vi "Generate Event.vi"(4 "Error In":errorcluster, 5 "Response Notifier":string, 6 "Data Buffer Depth":i32, 7 "Plugin Name":string) -> (0 "Error Out":errorcluster)   [LabVIEW 2015, in "Set Data Buffer Depth.lvlib"]
uses:
  Set Data Buffer Depth.lvlib
  _typedefs/Event Data.ctl
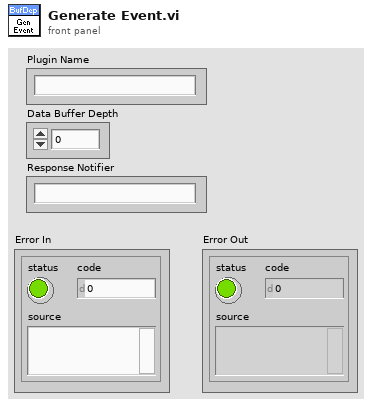
[diagram p1: front panel]
types:
  T1 = typedef "Set Data Buffer Depth.lvlib/Event Data.ctl" = cluster{"Plugin Name":string, "Data Buffer Depth":i32, "Response Notifier":string}
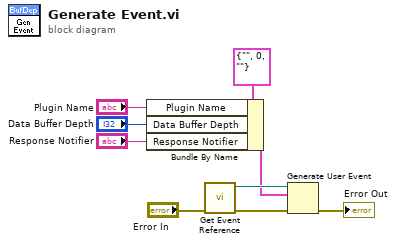
[diagram p0: block diagram]
diagram:
  n1 = Bundle By Name(cluster=T1 {"Plugin Name"="", "Data Buffer Depth"=0, "Response Notifier"=""} ("event data"), "Plugin Name"="Plugin Name", "Data Buffer Depth"="Data Buffer Depth", "Response Notifier"="Response Notifier") -> (w4:T1)
  n2 = call "Get Event Reference.vi"("error in (no error)"="Error In") -> ("error out"=w8:errorcluster, "Set Data Buffer Depth"=w7:refnum<user-event>)  [unwired: 5 in]
  n3 = Generate User Event(user event=w7, event data cluster=w4, error in=w8) -> (error out=→"Error Out":errorcluster)  [unwired: 1 in, 1 out]
